vi "Create Excel from Hidden.vi"(0 "DataFilePath":path, 2 "Controller List":T2(array[cluster]), 7 "TemplatePath":path, 11 "CMD Step":dbl format="%#_13g") -> (4 "Stat_Path":path, 6 "Data_Path":path, 8 "Spec_Path":path, 15 "Error Out":errorcluster)   [LabVIEW 2019]
uses:
  TypeDef/Controller Names.ctl
  <vilib>/Utility/file.llb/Read From Spreadsheet File (string).vi
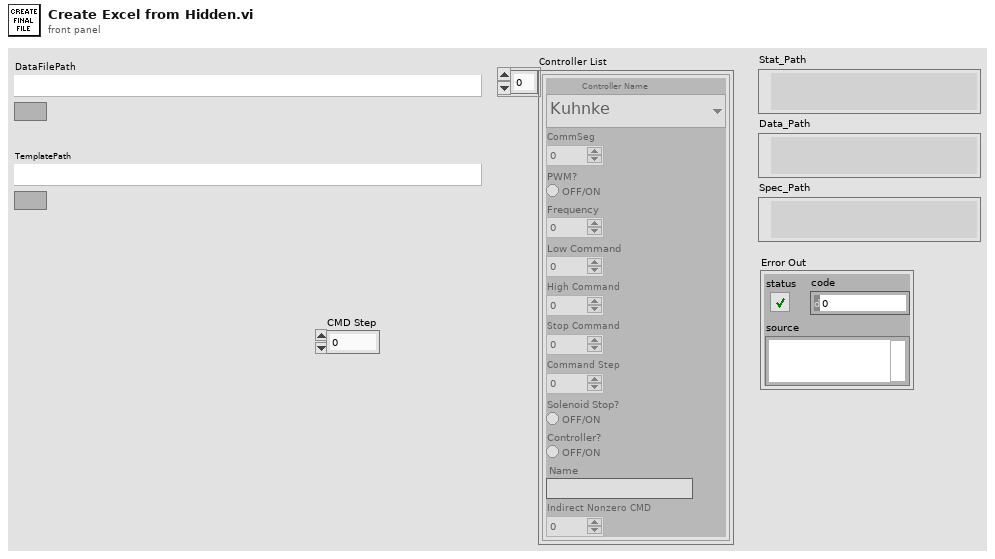
[diagram p1: front panel]
types:
  T1 = typedef "Controller Names.ctl" = enum16{"Kuhnke", "McLaren", "Helbako BLDC", "Conti", "Hella E4LMF", "Hella E4LMD", "Hella E4DCG 20mm", "Hella E4DCG 30mm", "Helbako (old)", "TI PWM", "PSA", "Hella Hyundai Gas", "Hella Hyundai Diesel", "8 Comm", "10 Comm", "8 Comm Hella FCA", "10 Comm Hella FCA", "8 Comm Omron", "10 Comm Omron", "8 Comm Nissan", "10 Comm Nissan", "8 Comm Hella (for FCA)", "Mazda BLDC"}
  T2 = cluster{"Controller Name":T1, "CommSeg":i32, "PWM?":bool, "Frequency":i32, "Low Command":dbl, "High Command":dbl, "Stop Command":dbl, "Command Step":dbl, "Solenoid Stop?":bool, "Controller?":bool, "Name":string, "Indirect Nonzero CMD":dbl}[]
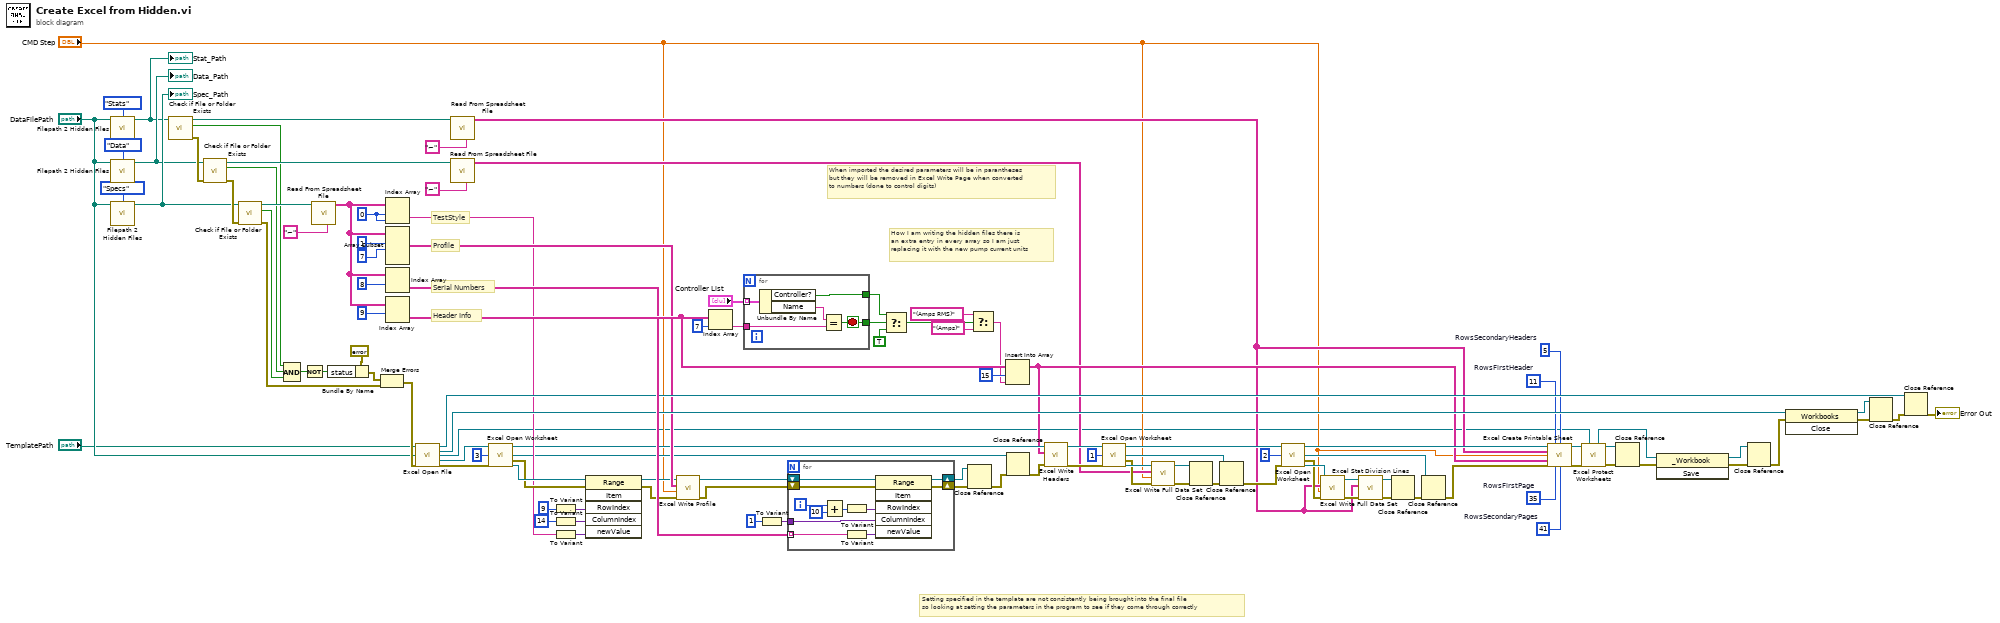
[diagram p0: block diagram]
diagram:
  w15 = 41  # RowsSecondaryPages
  w16 = 35  # RowsFirstPage
  w17 = 5  # RowsSecondaryHeaders
  w18 = 11  # RowsFirstHeader
  w80 = 0 ("index (row)")
  # "Setting specified in the template are not consistently being brought into the final file\nso looking at setting the parameters in the program to see if they come through correctly"
  # "When imported the desired parameters will be in parantheses\nbut they will be removed in Excel Write Page when converted\nto numbers (done to control digits)"
  # "How I am writing the hidden files there is\nan extra entry in every array so I am just\nreplacing it with the new pump current units"
  # "Header Info"
  # "Serial Numbers"
  # "Profile"
  # "TestStyle"
  n1 = call "Filepath 2 Hidden Files.vi"("DataFilePath"="DataFilePath", "Enum"=enum16{"Data", "Stats", "Specs"}."Stats") -> ("HiddenFilePath"=w85:path)  [unwired: 13 in]
  "Stat_Path" <- w85
  n2 = call "Filepath 2 Hidden Files.vi"("DataFilePath"="DataFilePath", "Enum"=enum16{"Data", "Stats", "Specs"}."Data") -> ("HiddenFilePath"=w86:path)  [unwired: 13 in]
  "Data_Path" <- w86
  n3 = call "Filepath 2 Hidden Files.vi"("DataFilePath"="DataFilePath", "Enum"=enum16{"Data", "Stats", "Specs"}."Specs") -> ("HiddenFilePath"=w87:path)  [unwired: 13 in]
  "Spec_Path" <- w87
  n4 = call <vilib>:"Check if File or Folder Exists.vi"("path"=w85) -> ("error out"=w96:errorcluster, "file or folder exists?"=w93:bool, "dup path"=w98:path)  [unwired: 8 in]
  n5 = call <vilib>:"Check if File or Folder Exists.vi"("error in (no error)"=w96, "path"=w86) -> ("error out"=w97:errorcluster, "file or folder exists?"=w94:bool, "dup path"=w100:path)  [unwired: 7 in]
  n6 = call <vilib>:"Check if File or Folder Exists.vi"("error in (no error)"=w97, "path"=w87) -> ("error out"=w42:errorcluster, "file or folder exists?"=w95:bool, "dup path"=w99:path)  [unwired: 7 in]
  n7 = Compound Arithmetic op=AND(w93, w94, w95) -> (w92:bool)
  n8 = Not(x=w92) -> (.not. x?=w90:bool)
  n9 = call-poly <vilib>:"Read From Spreadsheet File.vi"("delimiter (\\t)"="~" ("delimiter (\\t)"), "file path (dialog if empty)"=w99) -> ("all rows"=w108:string[][])  [unwired: 5 in, 4 out]
  n10 = Bundle By Name(cluster=errorcluster {"status"=FALSE, "code"=0, "source"=""} ("error constant"), "status"=w90) -> (w89:errorcluster)
  n11 = Merge Errors(w89, w42) -> (w41:errorcluster)
  n12 = Index Array(array=w108, index (row)=w80, index (col)=w80) -> (element=w32:string)
  n13 = Array Subset(array=w108, index (row)=1 ("index"), length (row)=7 ("length")) -> (w34:string[][])  [unwired: 2 in]
  n14 = Index Array(array=w108, index (row)=8) -> (element=w67:string[])  [unwired: 1 in]
  n15 = Index Array(array=w108, index (row)=9) -> (element=w70:string[])  [unwired: 1 in]
  n16 = call "Excel Open File.vi"("TemplatePath"="TemplatePath", "DataFilePath"="DataFilePath", "Error In"=w41) -> ("Excel Ref Out"=w40:refnum<k7>, "WorkbookS Ref Out"=w39:refnum<k7>, "Workbook Ref Out"=w2:refnum<k7>, "Sheets Ref Out"=w38:refnum<k7>, "Error Out"=w37:errorcluster)  [unwired: 8 in]
  n17 = call-poly <vilib>:"Read From Spreadsheet File.vi"("delimiter (\\t)"="~" ("delimiter (\\t)"), "file path (dialog if empty)"=w98) -> ("all rows"=w14:string[][])  [unwired: 5 in, 4 out]
  n18 = call-poly <vilib>:"Read From Spreadsheet File.vi"("delimiter (\\t)"="~" ("delimiter (\\t)"), "file path (dialog if empty)"=w100) -> ("all rows"=w13:string[][])  [unwired: 5 in, 4 out]
  n19 = call "Excel Open Worksheet.vi"("Sheets Ref In"=w38, "Sheet#"=3, "Error In"=w37) -> ("Sheets Ref Out"=w31:refnum<k7>, "Worksheet Ref Out"=w30:refnum<k7>, "Error Out"=w35:errorcluster, "Cells Ref Out"=w36:refnum<k7>)  [unwired: 9 in]
  n20 = To Variant(anything=9) -> (Variant=w84:variant)
  n21 = To Variant(anything=14) -> (Variant=w81:variant)
  n22 = To Variant(anything=w32) -> (Variant=w82:variant)
  n23 = invoke class="Range" method="Item"(reference=w36, error in=w35, "RowIndex"=w84, "ColumnIndex"=w81, "newValue"=w82) -> (reference out=w12:refnum<k7>, error out=w33:errorcluster)  [unwired: 1 in, 4 out]
  n24 = call "Excel Write Profile.vi"("Error In"=w33, "CMD Step"="CMD Step", "Profile"=w34, "Cells Ref In"=w12) -> ("Error Out"=w29:errorcluster, "Cells Ref Out"=w28:refnum<k7>)  [unwired: 6 in]
  n25 = Index Array(array=w70, index=7) -> (element=w77:string)
  n26 = for {
    tunnel: "Controller List" -> [w119] mode=indexing
    tunnel: w77 -> [w117]
    tunnel: [w116] -> w76
    tunnel: [w115] -> w72
    stop <- w115 stop-if-true
    n27 = Unbundle By Name(w119) -> ("Controller?"=w116:bool, "Name"=w118:string)
    n28 = Equal?(x=w118, y=w117) -> (x = y?=w115:bool)
  }
  n29 = To Variant(anything=1 ("y")) -> (Variant=w101:variant)
  n30 = for {
    tunnel: w67 -> [w127] mode=indexing
    tunnel: w101 -> [w123]
    shift-right: [w121] -> w66
    shift-left: w28 -> [w128]
    shift-right: [w120] -> w65
    shift-left: w29 -> [w122]
    i -> [w125]
    n31 = Add(x=w125, y=10) -> (x+y=w124:i32)
    n32 = To Variant(anything=w124) -> (Variant=w130:variant)
    n33 = To Variant(anything=w127) -> (Variant=w129:variant)
    n34 = invoke class="Range" method="Item"(reference=w128, error in=w122, "RowIndex"=w130, "ColumnIndex"=w123, "newValue"=w129) -> (reference out=w121:refnum<k7>, error out=w120:errorcluster)  [unwired: 1 in, 4 out]
  }
  n35 = Select(t=w76, s=w72, f=TRUE) -> (s? t:f=w71:bool)
  n36 = Close Reference(reference=w66, error in (no error)=w65) -> (error out=w61:errorcluster)
  n37 = Select(t="(Amps RMS)", s=w71, f="(Amps)") -> (s? t:f=w68:string)
  n38 = Insert Into Array(array=w70, index=15, new element=w68) -> (w19:string[])
  n39 = Close Reference(reference=w30, error in (no error)=w61) -> (error out=w44:errorcluster)
  n40 = call "Excel Write Headers.vi"("Error In"=w44, "Header Info"=w19, "Sheets Ref In"=w31) -> ("Error Out"=w26:errorcluster, "Sheets Ref Out"=w27:refnum<k7>)  [unwired: 7 in]
  n41 = call "Excel Open Worksheet.vi"("Sheets Ref In"=w27, "Sheet#"=1, "Error In"=w26) -> ("Sheets Ref Out"=w47:refnum<k7>, "Worksheet Ref Out"=w51:refnum<k7>, "Error Out"=w52:errorcluster, "Cells Ref Out"=w53:refnum<k7>)  [unwired: 9 in]
  n42 = call "Excel Write Full Data Set.vi"("Error In"=w52, "CMD Step"="CMD Step", "Data In"=w13, "Cells Ref In"=w53) -> ("Error Out"=w60:errorcluster, "Cells Ref Out"=w59:refnum<k7>)  [unwired: 6 in]
  n43 = Close Reference(reference=w59, error in (no error)=w60) -> (error out=w62:errorcluster)
  n44 = Close Reference(reference=w51, error in (no error)=w62) -> (error out=w46:errorcluster)
  n45 = call "Excel Open Worksheet.vi"("Sheets Ref In"=w47, "Sheet#"=2, "Error In"=w46) -> ("Sheets Ref Out"=w25:refnum<k7>, "Worksheet Ref Out"=w48:refnum<k7>, "Error Out"=w49:errorcluster, "Cells Ref Out"=w50:refnum<k7>)  [unwired: 9 in]
  n46 = call "Excel Write Full Data Set.vi"("Error In"=w49, "CMD Step"="CMD Step", "Data In"=w14, "Cells Ref In"=w50) -> ("Error Out"=w55:errorcluster, "Cells Ref Out"=w56:refnum<k7>)  [unwired: 6 in]
  n47 = call "Excel Stat Division Lines.vi"("Error In"=w55, "Data In"=w14, "Cells Ref In"=w56) -> ("Error Out"=w57:errorcluster, "Cells Ref Out"=w58:refnum<k7>)  [unwired: 7 in]
  n48 = Close Reference(reference=w58, error in (no error)=w57) -> (error out=w63:errorcluster)
  n49 = Close Reference(reference=w48, error in (no error)=w63) -> (error out=w24:errorcluster)
  n50 = call "Excel Create Printable Sheet.vi"("Sheets Ref In"=w25, "RowsFirstHeader"=w18, "RowsHeadersAfter"=w17, "Stat Array"=w14, "CMD Step"="CMD Step", "HeaderInfo"=w19, "Error In"=w24, "RowsFirstPage"=w16, "RowsPagesAfter"=w15) -> ("Sheets Ref Out"=w23:refnum<k7>, "Error Out"=w22:errorcluster)  [unwired: 5 in]
  n51 = call "Excel Protect Worksheets.vi"("Sheets Ref In"=w23, "Workbook Ref In"=w2, "Error In"=w22) -> ("Workbook Ref Out"=w1:refnum<k7>, "Sheets Ref Out"=w21:refnum<k7>, "Error Out"=w20:errorcluster)  [unwired: 10 in]
  n52 = Close Reference(reference=w21, error in (no error)=w20) -> (error out=w64:errorcluster)
  n53 = invoke class="_Workbook" method="Save"(reference=w1, error in=w64) -> (reference out=w6:refnum<k7>, error out=w9:errorcluster)  [unwired: 1 in, 1 out]
  n54 = Close Reference(reference=w6, error in (no error)=w9) -> (error out=w8:errorcluster)
  n55 = invoke class="Workbooks" method="Close"(reference=w39, error in=w8) -> (reference out=w7:refnum<k7>, error out=w10:errorcluster)  [unwired: 1 in, 1 out]
  n56 = Close Reference(reference=w7, error in (no error)=w10) -> (error out=w11:errorcluster)
  n57 = Close Reference(reference=w40, error in (no error)=w11) -> (error out=→"Error Out":errorcluster)
